vi "Call Vaa3D.vi"(7 "Vaa3D path":path, 8 "error in (no error)":errorcluster, 9 "spacing_between_points":dbl, 10 "Call_Vaa3D":bool, 11 "Z-stack folder path":path) -> (0 "error out":errorcluster)   [LabVIEW 2017]
panel:
  # "E:\\Vaa3D\\Vaa3D_V3.497_Windows_MSVC_64bit"
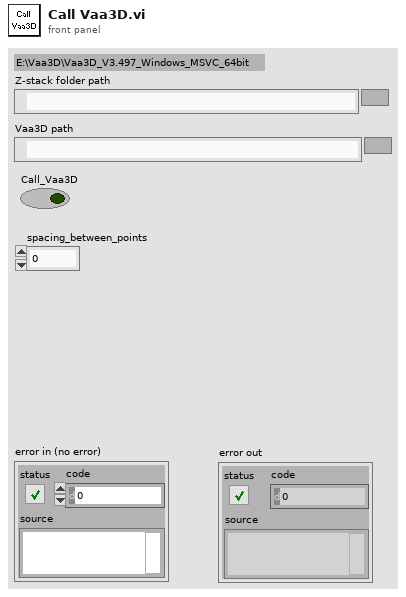
[diagram p1: front panel]
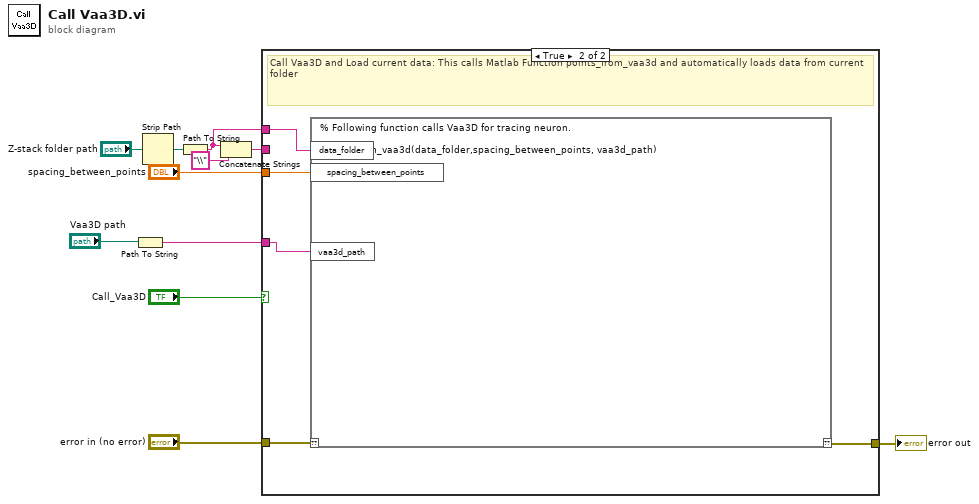
[diagram p0: block diagram]
diagram:
  n1 = Path To String(path="Vaa3D path") -> (string=w2:string)
  n2 = Strip Path(path="Z-stack folder path") -> (stripped path=w6:path)  [unwired: 1 out]
  n3 = Path To String(path=w6) -> (string=w1:string)
  n4 = Concatenate Strings(w1, "\\" ("string")) -> (w5:string)
  n5 = case shown="True" "Call_Vaa3D" {
    tunnel: "spacing_between_points" -> [_ w17]
    tunnel: w5 -> [_ _]
    tunnel: [w12 w16] -> w8
    tunnel: "error in (no error)" -> [w12 w15]
    tunnel: w2 -> [_ w14]
    tunnel: w1 -> [_ w13]
    frame False {
    }
    frame True {
      # "Call Vaa3D and Load current data: This calls Matlab Function points_from_vaa3d and automatically loads data from current folder"
      n6 = script code="% Following function calls Vaa3D for tracing neuron.\n\npoints_from_vaa3d(data_folder,spacing_between_points, vaa3d_path)"("??"=w15, "spacing_between_points"=w17, "data_folder"=w13, "vaa3d_path"=w14) -> ("??"=w16:errorcluster)
    }
  }
  "error out" <- w8
